vi "InitMixerMessage.vi"(9 "value":dbl, 10 "Param":T1, 11 "Operation":T2) -> (3 "MixerMessage out":refnum<class "MixerMessage.lvclass">)   [LabVIEW 2013, in "MixerMessage.lvclass"]
uses:
  MixerMessage.lvclass
  MixerOperation.ctl
  MixerParam.ctl
  MixerMessage.lvclass/MixerMessage.ctl
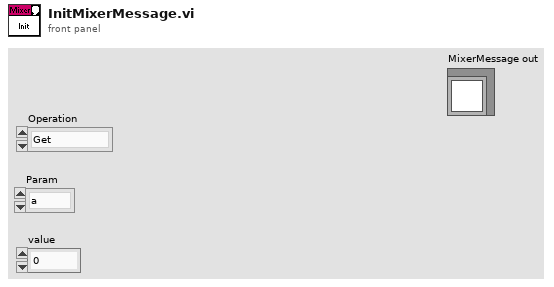
[diagram p1: front panel]
types:
  T1 = typedef "MixerMessage.lvclass/MixerParam.ctl" = enum16{"a", "b", "fm"}
  T2 = typedef "MixerMessage.lvclass/MixerOperation.ctl" = enum16{"Get", "Set"}
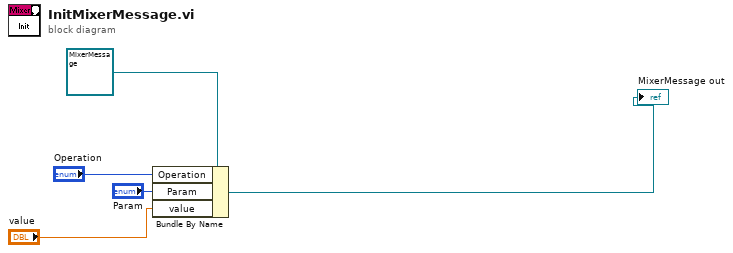
[diagram p0: block diagram]
diagram:
  n1 = Bundle By Name(cluster=refnum<class "MixerMessage.lvclass"> refnum ("MixerMessage out"), "Operation"="Operation", "Param"="Param", "value"="value") -> (→"MixerMessage out":refnum<class "MixerMessage.lvclass">)
